vi "Log Failed.vi"(7 "RESULTADO":string, 8 "Case number":i32, 9 "Image In":T1, 10 "Boolean":bool, 11 "GABARITO":string) -> ()   [LabVIEW 2016, in "MVP02 Custom Device.lvlib"]
uses:
  MVP02 Custom Device.lvlib
  <vilib>/vision/Image Controls.llb/IMAQ Image.ctl
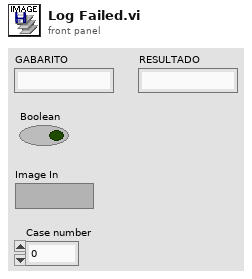
[diagram p1: front panel]
types:
  T1 = typedef "IMAQ Image.ctl" = refnum<image>
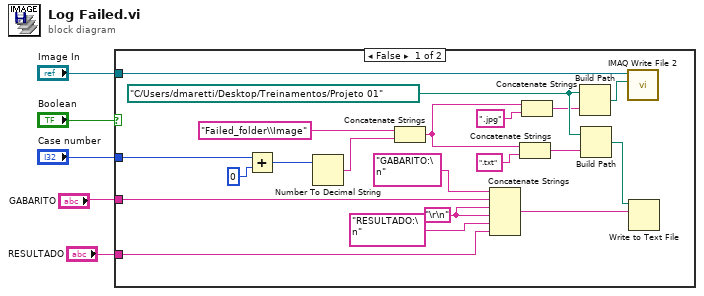
[diagram p0: block diagram]
diagram:
  n1 = case shown="False" "Boolean" {
    tunnel: "Image In" -> [w25 _]
    tunnel: "Case number" -> [w19 _]
    tunnel: "GABARITO" -> [w11 _]
    tunnel: "RESULTADO" -> [w8 _]
    frame False {
      w6 = "\r\n"
      w17 = path "C:/Users/dmaretti/Desktop/Treinamentos/Projeto 01" ("base path")
      n2 = Add(x=w19, y=0) -> (x+y=w21:i32)
      n3 = Number To Decimal String(number=w21) -> (decimal integer string=w22:string)  [unwired: 1 in]
      n4 = Concatenate Strings("Failed_folder\\Image" ("name or relative path"), w22) -> (w13:string)
      n5 = Concatenate Strings("GABARITO:\n" ("string"), w11, w6, w6, "RESULTADO:\n" ("string"), w8) -> (w10:string)
      n6 = Concatenate Strings(w13, ".txt" ("string")) -> (w12:string)
      n7 = Concatenate Strings(w13, ".jpg" ("string")) -> (w16:string)
      n8 = Build Path(base path=w17, name or relative path=w16) -> (appended path=w24:path)
      n9 = Build Path(base path=w17, name or relative path=w12) -> (appended path=w15:path)
      n10 = call-poly "IMAQ Write File 2"("File Path"=w24, "Image"=w25) -> ()  [unwired: 8 in, 2 out]
      n11 = Write to Text File(file (use dialog)=w15, text=w10) -> ()  [unwired: 2 in, 3 out]
    }
    frame True {
    }
  }
